vi "Multi Points Volt to physical quantity.vi"(6 "precision (6)":u8=3, 7 "Single(T)":bool, 8 "error out":errorcluster, 9 "Real Volt Single":dbl, 10 "Real Volt":dbl[](array[numeric]), 11 "Calibration Kb&Volts":T1) -> (0 "error out":errorcluster, 2 "physical quantity Single":dbl, 3 "physical quantity":dbl[](array[numeric]))   [LabVIEW 2017, in "SQLite.lvclass"]
doc: "多点校准模块。\n2015-07-12 15:11:47\n蒋松\njiangsong@outlook.com"
uses:
  SQLite.lvclass
  Calibration Kb and Volt.ctl
  Calibration K and b Array.ctl
  Calibration K and b.ctl
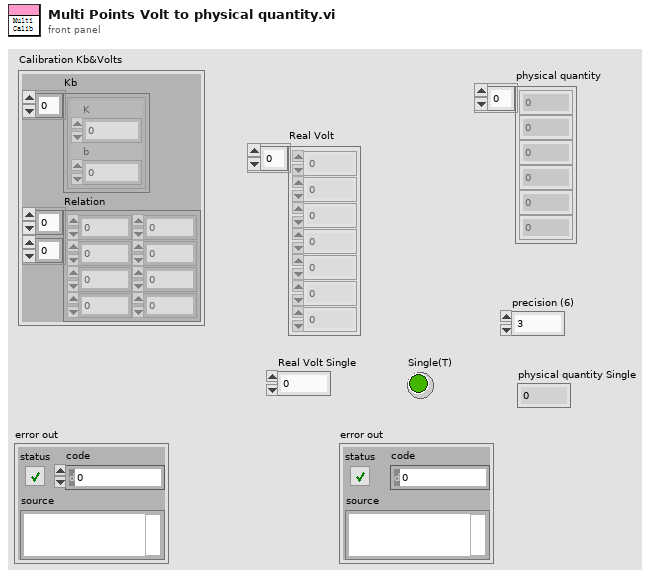
[diagram p1: front panel]
types:
  T1 = typedef "SQLite.lvclass/Calibration Kb and Volt.ctl" = cluster{"Kb":T2, "Relation":dbl[][]}
  T2 = typedef "SQLite.lvclass/Calibration K and b Array.ctl" = T3[]
  T3 = typedef "SQLite.lvclass/Calibration K and b.ctl" = cluster{"K":dbl, "b":dbl}
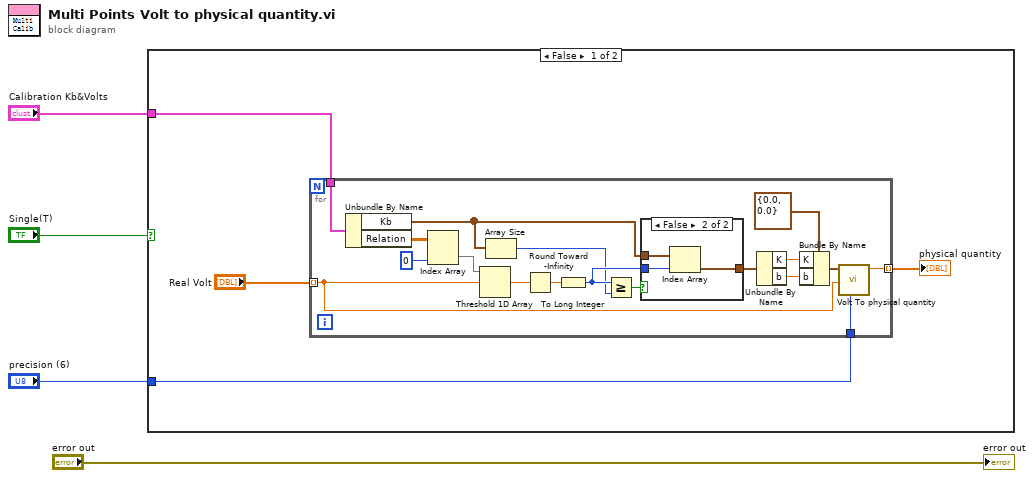
[diagram p0: block diagram]
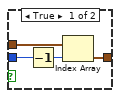
[diagram p2: hidden frame]
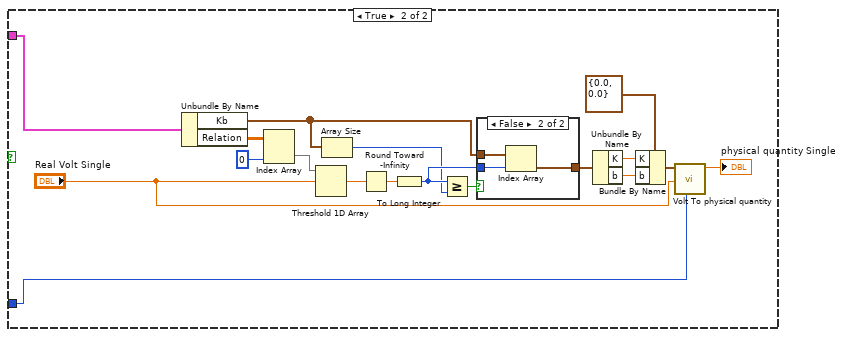
[diagram p3: hidden frame]
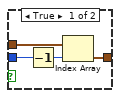
[diagram p4: hidden frame]
diagram:
  n1 = case shown="False" "Single(T)" {
    tunnel: "precision (6)" -> [w8 w49]
    tunnel: "Calibration Kb&Volts" -> [w7 w50]
    frame False {
      n2 = for {
        tunnel: w7 -> [w21]
        tunnel: "Real Volt" -> [w20] mode=indexing
        tunnel: [w18] -> w6 mode=indexing
        tunnel: w8 -> [w10]
        n3 = Unbundle By Name(w21) -> ("Kb"=w19:T2, "Relation"=w17:dbl[][])
        n4 = Index Array(array=w17, index (col)=0 ("disabled index (col)")) -> (element=w16:dbl[])  [unwired: 1 in]
        n5 = Threshold 1D Array(2:w20, 3:w16) -> (0:w22:dbl)  [unwired: 1 in]
        n6 = Array Size(array=w19) -> (size(s)=w23:i32)
        n7 = Round Toward -Infinity(1:w22) -> (0:w25:dbl)
        n8 = To Long Integer(number=w25) -> (32bit integer=w26:i32)
        n9 = Greater Or Equal?(x=w26, y=w23) -> (x >= y?=w24:bool)
        n10 = case shown="False" w24 {
          tunnel: w19 -> [w30 w33]
          tunnel: w26 -> [w28 w32]
          tunnel: [w29 w31] -> w13
          frame True {
            n11 = Decrement(x=w28) -> (x-1=w27:i32)
            n12 = Index Array(array=w30, index=w27) -> (element=w29:T3)
          }
          frame False {
            n13 = Index Array(array=w33, index=w32) -> (element=w31:T3)
          }
        }
        n14 = Unbundle By Name(w13) -> ("K"=w12:dbl, "b"=w11:dbl)
        n15 = Bundle By Name(cluster=T3 {"K"=0.0, "b"=0.0} ("Calibration"), "K"=w12, "b"=w11) -> (w14:T3)
        n16 = call "Volt To physical quantity.vi"("precision (6)"=w10, "Volt Input"=w20, "Calibration"=w14) -> ("physical quantity"=w18:dbl)  [unwired: 8 in]
      }
      "physical quantity" <- w6
    }
    frame True {
      n17 = Unbundle By Name(w50) -> ("Kb"=w43:T2, "Relation"=w42:dbl[][])
      n18 = Index Array(array=w42, index (col)=0 ("disabled index (col)")) -> (element=w41:dbl[])  [unwired: 1 in]
      n19 = Threshold 1D Array(2:"Real Volt Single", 3:w41) -> (0:w44:dbl)  [unwired: 1 in]
      n20 = Array Size(array=w43) -> (size(s)=w45:i32)
      n21 = Round Toward -Infinity(1:w44) -> (0:w47:dbl)
      n22 = To Long Integer(number=w47) -> (32bit integer=w48:i32)
      n23 = Greater Or Equal?(x=w48, y=w45) -> (x >= y?=w46:bool)
      n24 = case shown="False" w46 {
        tunnel: w43 -> [w55 w58]
        tunnel: w48 -> [w53 w57]
        tunnel: [w54 w56] -> w38
        frame True {
          n25 = Decrement(x=w53) -> (x-1=w52:i32)
          n26 = Index Array(array=w55, index=w52) -> (element=w54:T3)
        }
        frame False {
          n27 = Index Array(array=w58, index=w57) -> (element=w56:T3)
        }
      }
      n28 = Unbundle By Name(w38) -> ("K"=w37:dbl, "b"=w36:dbl)
      n29 = Bundle By Name(cluster=T3 {"K"=0.0, "b"=0.0} ("Calibration"), "K"=w37, "b"=w36) -> (w39:T3)
      n30 = call "Volt To physical quantity.vi"("precision (6)"=w49, "Volt Input"="Real Volt Single", "Calibration"=w39) -> ("physical quantity"=→"physical quantity Single":dbl)  [unwired: 8 in]
    }
  }
  "error out" <- "error out"
